vi "SetAllowedViInfomation.vi"(8 "error in (no error)":errorcluster caption="错误输入（无错误）", 11 "PanelRootNode 输入":refnum<class "PanelRootNode.lvclass"> caption="DNL_LabVIEW Object in") -> (0 "error out":errorcluster caption="错误输出", 1 "ViPath":path[](array[path]), 2 "ViAlias":string[](array[string]), 3 "PanelRootNode 输出":refnum<class "PanelRootNode.lvclass"> caption="DNL_LabVIEW Object out")   [LabVIEW 2016, in "PanelRootNode.lvclass"]
uses:
  PanelRootNode.lvclass
  PanelDataNode/PanelDataNode.lvclass
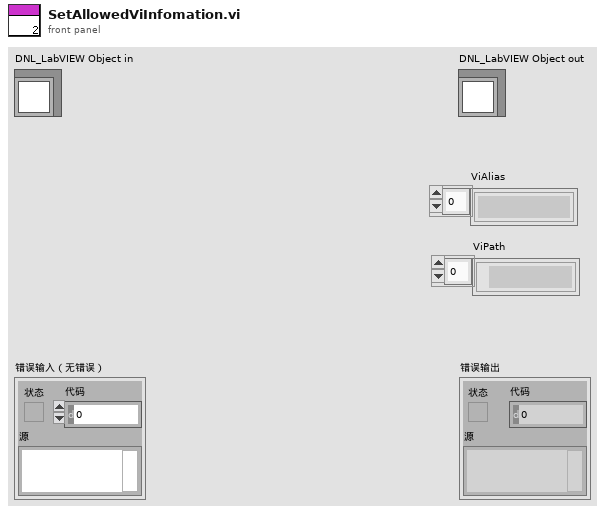
[diagram p1: front panel]
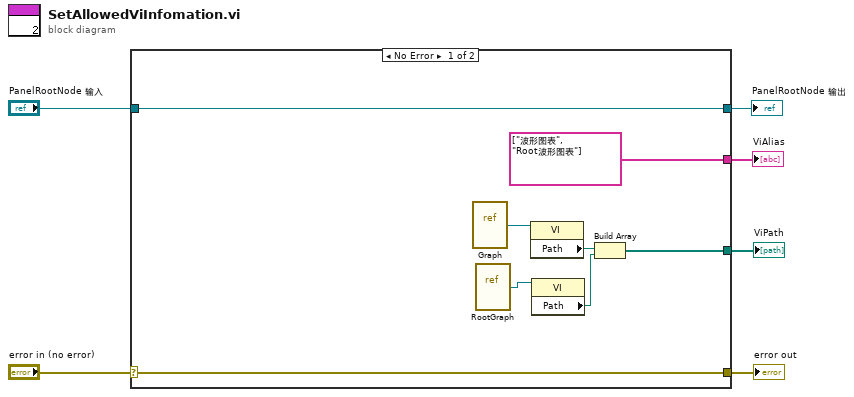
[diagram p0: block diagram]
diagram:
  n1 = case shown="No Error" "error in (no error)" {
    selector: "error in (no error)" -> [w13 w16]
    tunnel: [w13 w16] -> w5
    tunnel: [w14 w15] -> w3
    tunnel: "PanelRootNode 输入" -> [w14 w15]
    tunnel: [string[] ["波形图表", "Root波形图表"] ("Allowed VI Alias") _] -> w2
    tunnel: [w7 _] -> w1
    frame No Error {
      n2 = vi-ref "Graph.vi"() -> (w8:refnum<vi>)
      n3 = vi-ref "RootGraph.vi"() -> (w10:refnum<vi>)
      n4 = property class="VI"(reference=w8) -> ("Path"=w9:path)  [unwired: 1 in, 2 out]
      n5 = property class="VI"(reference=w10) -> ("Path"=w11:path)  [unwired: 1 in, 2 out]
      n6 = Build Array(w9, w11) -> (w7:path[])
    }
    frame Error {
    }
  }
  "error out" <- w5
  "PanelRootNode 输出" <- w3
  "ViAlias" <- w2
  "ViPath" <- w1
